vi "Construct Recursive JSON Serializable.vi"(5 "Recursive JSON Serializable in":refnum<class "Recursive JSON Serializable.lvclass">, 8 "error in (no error)":errorcluster, 10 "Recursion Level":u8) -> (0 "error out":errorcluster, 3 "Recursive JSON Serializable":refnum<class "Recursive JSON Serializable.lvclass">)   [LabVIEW 2017, in "JSON Serializable Serializer Tests.lvlib" / "Recursive JSON Serializable.lvclass"]
uses:
  Recursive JSON Serializable.lvclass
  Recursive JSON Serializable.lvclass/Recursive JSON Serializable.ctl
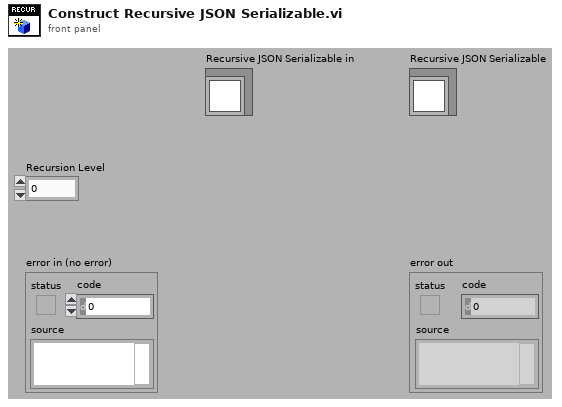
[diagram p1: front panel]
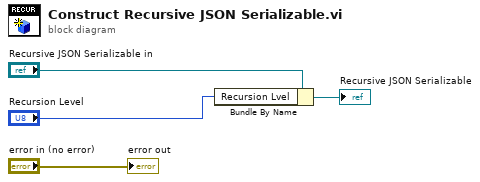
[diagram p0: block diagram]
diagram:
  n1 = Bundle By Name(cluster="Recursive JSON Serializable in", "Recursion Lvel"="Recursion Level") -> (→"Recursive JSON Serializable":refnum<class "Recursive JSON Serializable.lvclass">)
  "error out" <- "error in (no error)"
